vi "MessageBase.getNamesAndValues.vi"(8 "error in (no error)":errorcluster, 10 "Cluster":cluster{}, 11 "MessageBase in":refnum<class "MessageBase.lvclass">) -> (0 "error out":errorcluster, 2 "Array":cluster{"Value":variant, "Text":string}[](array[cluster]), 3 "MessageBase out":refnum<class "MessageBase.lvclass">)   [LabVIEW 2020]
uses:
  MessageBase.lvclass
  Trade/TradeBase.Parameters.ctl
  Trade/TradeBase.lvclass
panel:
  in  "TradeBase.Parms":T1={"Time Offset"=447000, "Order Id"="ORID0001", "Quantity"=20000, "Symbol"="AAPL", "Side Indicator"="B", "Price"=0.905, "Execution Id"="EXE_ID_1"}
  in  "Cluster 2":cluster{}
  out "Variant":variant
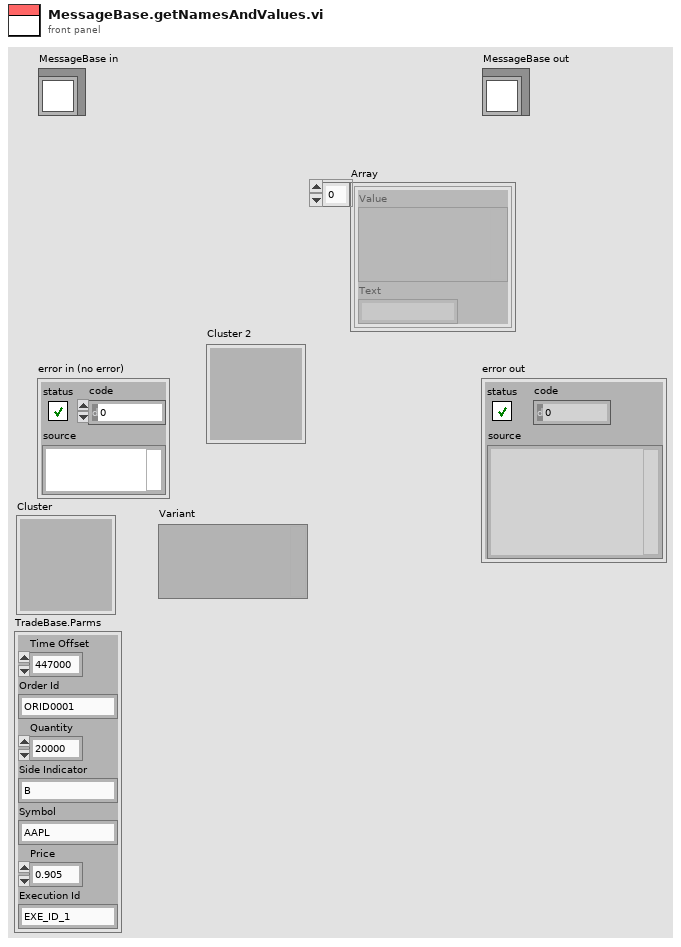
[diagram p1: front panel]
types:
  T1 = typedef "TradeBase.lvclass/TradeBase.Parameters.ctl" = cluster{"Time Offset":u32, "Order Id":string, "Quantity":u32, "Symbol":string, "Side Indicator":string, "Price":dbl, "Execution Id":string}
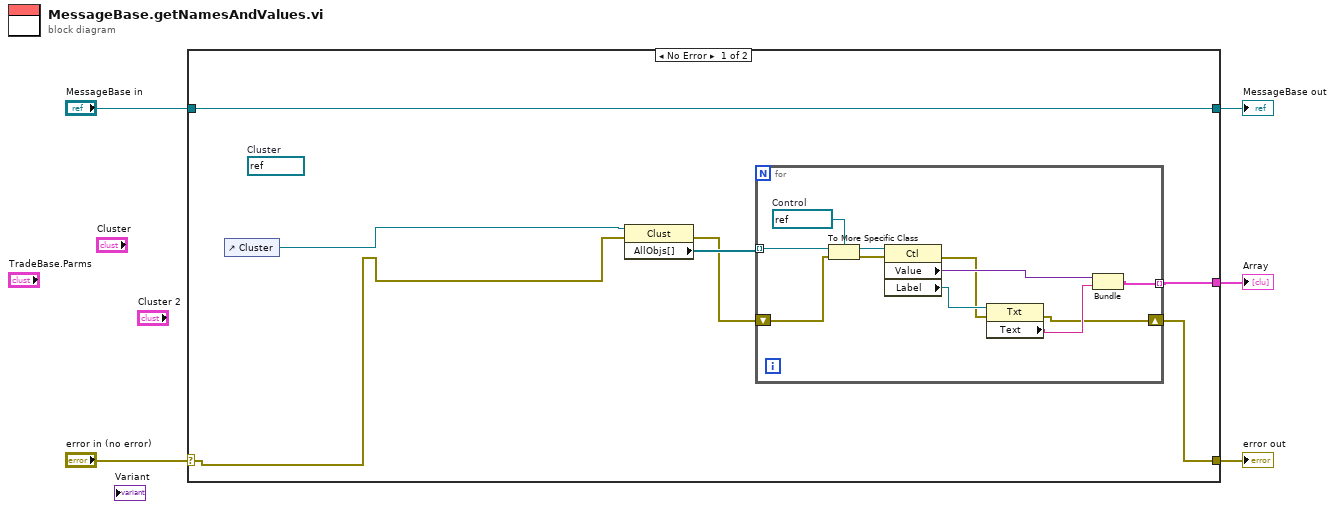
[diagram p0: block diagram]
diagram:
  n1 = case shown="No Error" "error in (no error)" {
    selector: "error in (no error)" -> [w6 w25]
    tunnel: [w8 w25] -> w4
    tunnel: [w12 w24] -> w2
    tunnel: "MessageBase in" -> [w12 w24]
    tunnel: [w9 _] -> w1
    frame No Error {
      (unwired) refnum<vi> refnum  # Cluster
      n2 = control-ref of="Cluster"() -> (w7:refnum<vi>)
      n3 = property class="Clust"(reference=w7, error in=w6) -> (error out=w10:errorcluster, "AllObjs[]"=w11:refnum<vi>[])  [unwired: 1 out]
      n4 = for {
        tunnel: w11 -> [w23] mode=indexing
        tunnel: [w16] -> w9 mode=indexing
        shift-right: [w13] -> w8
        shift-left: w10 -> [w15]
        w22 = refnum<vi> refnum  # Control
        n5 = To More Specific Class(target class=w22, reference=w23, error in=w15) -> (specific class reference=w21:refnum<vi>, error out=w20:errorcluster)
        n6 = property class="Ctl"(reference=w21, error in=w20) -> (error out=w14:errorcluster, "Value"=w19:variant, "Label"=w18:refnum<vi>)  [unwired: 1 out]
        n7 = property class="Txt"(reference=w18, error in=w14) -> (error out=w13:errorcluster, "Text"=w17:string)  [unwired: 1 out]
        n8 = Bundle("Value"=w19, "Text"=w17) -> (w16:cluster{"Value":variant, "Text":string})  [unwired: 1 in]
      }
    }
    frame Error {
    }
  }
  "error out" <- w4
  "MessageBase out" <- w2
  "Array" <- w1
